vi "Test MQTT-3.1.3-3.vi"(8 "error in (no error)":errorcluster) -> (0 "error out":errorcluster)   [LabVIEW 2013]
uses:
  source/Control Packets/CONNECT/ConnectFlags -- cluster.ctl
  source/Control Packets/ControlPacket/ControlPacket.lvclass/ControlPacket.ctl
  <vilib>/addons/_JKI Toolkits/Caraya/classes/Assert/Assert Equal Value_Variant.vi
  source/Control Packets/CONNECT/CONNECT.lvclass
  <vilib>/addons/_JKI Toolkits/Caraya/classes/Test/Test.lvclass
  <vilib>/addons/_JKI Toolkits/Caraya/classes/Assert/Assert.lvclass
  source/Control Packets/ControlPacket/ControlPacket.lvclass
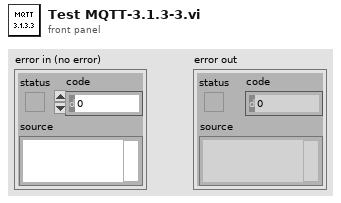
[diagram p1: front panel]
types:
  T1 = cluster{"Will Topic":string, "Will Message":string, "Username":string, "Password":string}
  T2 = typedef "CONNECT.lvclass/ConnectFlags -- cluster.ctl" = cluster{"Reserved":bool, "Clean Session":bool, "Will Flag":bool, "Will QoS 1":bool, "Will QoS 2":bool, "Will Retain":bool, "Password Flag":bool, "User Name Flag":bool}
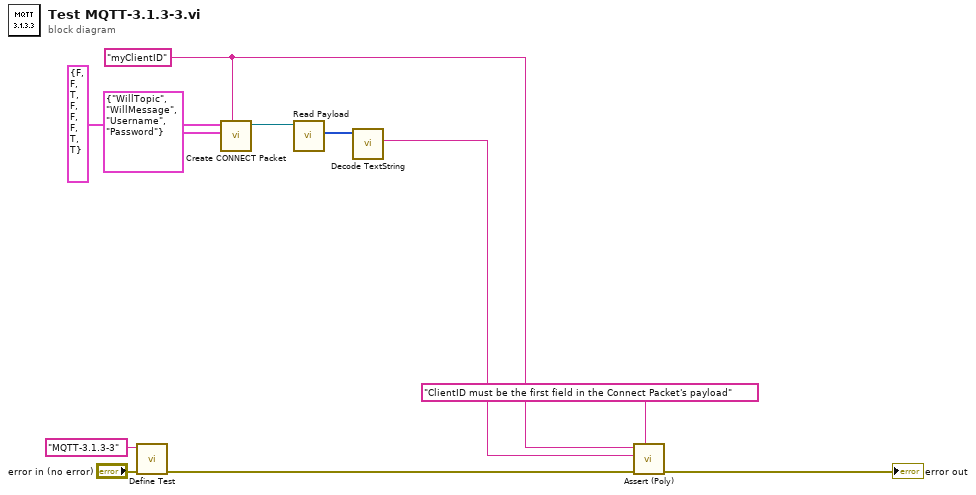
[diagram p0: block diagram]
diagram:
  w2 = "myClientID" ("Client ID (empty: generate new)")
  n1 = call <vilib>:"Define Test.vi"("error in (no error)"="error in (no error)", "Label (VI Title)"="MQTT-3.1.3-3") -> ("error out"=w8:errorcluster)  [unwired: 9 in]
  n2 = call "Create CONNECT Packet.vi"("Client ID (empty: generate new)"=w2, "Payload"=T1 {"Will Topic"="WillTopic", "Will Message"="WillMessage", "Username"="Username", "Password"="Password"}, "Connect Flags"=T2 {"Reserved"=FALSE, "Clean Session"=FALSE, "Will Flag"=TRUE, "Will QoS 1"=FALSE, "Will QoS 2"=FALSE, "Will Retain"=FALSE, "Password Flag"=TRUE, "User Name Flag"=TRUE}) -> ("CONNECT"=w3:refnum<class "CONNECT.lvclass">)  [unwired: 7 in, 1 out]
  n3 = call "Read Payload.vi"("ControlPacket in"=w3) -> ("Payload"=w4:u8[])  [unwired: 9 in, 1 out]
  n4 = call "Decode TextString.vi"("Length-Prefixed Field"=w4) -> ("Text String"=w1:string)  [unwired: 8 in, 2 out]
  n5 = call-poly <vilib>:"Assert (Poly).vi"("Label"="ClientID must be the first field in the Connect Packet's payload", "error in (no error)"=w8, "Y"=w1, "X"=w2) -> ("error out"=→"error out":errorcluster)  [unwired: 7 in]
